vi "Teardown.vi"(7 "Actor in":refnum<class "Actor.lvclass">, 11 "jettl State in":refnum<class "jettl State.lvclass">) -> (2 "Teardown?":bool, 5 "Actor out":refnum<class "Actor.lvclass">)   [LabVIEW 2021, in "jettl.lvlib" / "jettl State.lvclass"]
uses:
  jettl State.lvclass
  Actor/Actor.lvclass
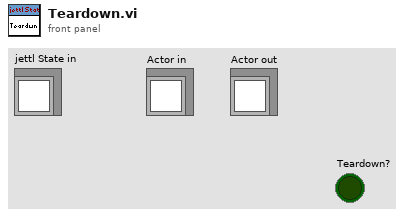
[diagram p1: front panel]
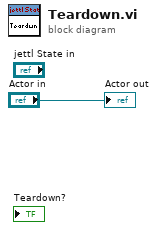
[diagram p0: block diagram]
diagram:
  "Actor out" <- "Actor in"
